vi "Binary Terminal.vi"() -> ()   [LabVIEW 2019]
uses:
  <vilib>/Instr/_visa.llb/VISA Configure Serial Port (Instr).vi
panel:
  in  "Value":dbl=10.0
  in  "CMD":u8(ring) items=["Request Data"=0, "Set Max"=2, "Set Min"=3]
  in  "Send":bool
  out "Chart":dbl(graph)
  out "error out":errorcluster
  in  "stop":bool
  in  "VISA resource name":refnum<visa-resource-name>
  # "To test this code, use a NULL Modem cable and use Binary Instrument.vi to act as the instrument"
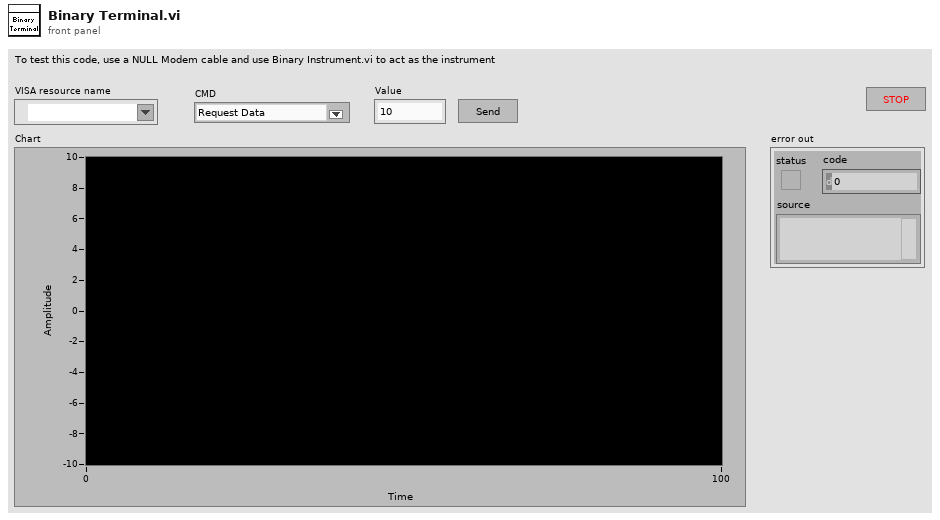
[diagram p1: front panel]
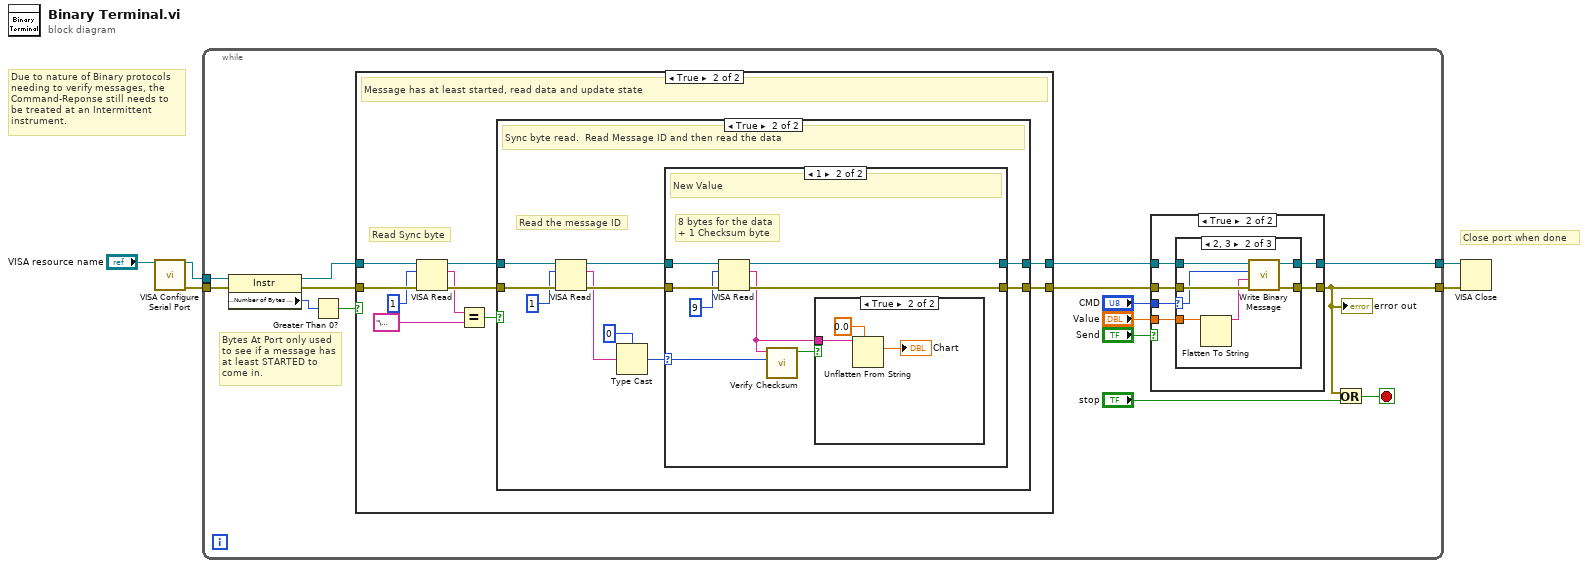
[diagram p0: block diagram]
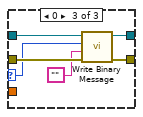
[diagram p4: hidden frame]
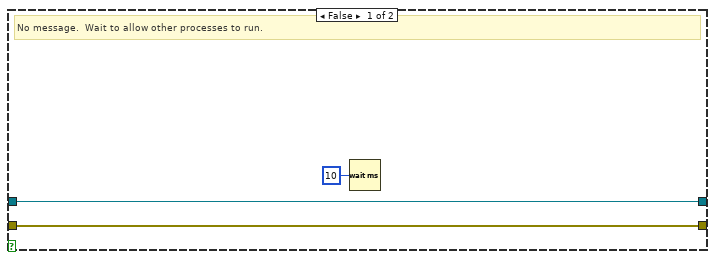
[diagram p5: hidden frame]
diagram:
  # "Due to nature of Binary protocols\nneeding to verify messages, the\nCommand-Reponse still needs to \nbe treated at an Intermittent\ninstrument."
  # "Close port when done"
  n1 = call-poly "VISA Configure Serial Port"("VISA resource name"="VISA resource name") -> ("VISA resource name out"=w1:refnum<visa-resource-name>, "error out"=w4:errorcluster)  [unwired: 13 in]
  n2 = while {
    tunnel: w4 -> [w20]
    tunnel: w1 -> [w16]
    tunnel: [w7] -> w2
    tunnel: [w18] -> w5
    stop <- w12 stop-if-true
    # "Bytes At Port only used\nto see if a message has\nat least STARTED to\ncome in."
    n3 = property class="Instr"(reference=w16, error in=w20) -> (reference out=w13:refnum<visa-resource-name>, error out=w19:errorcluster, "Serial Settings:Number of Bytes at Serial Port"=w15:u32)
    n4 = Greater Than 0?(x=w15) -> (x > 0?=w14:bool)
    n5 = case shown="True" w14 {
      tunnel: w19 -> [w46 w56]
      tunnel: w13 -> [w45 w53]
      tunnel: [w45 w47] -> w6
      tunnel: [w46 w54] -> w17
      frame False {
        # "No message.  Wait to allow other processes to run."
        n6 = Wait (ms)(milliseconds to wait=u32 10) -> ()  [unwired: 1 out]
      }
      frame True {
        # "Read Sync byte"
        # "Message has at least started, read data and update state"
        n7 = VISA Read(VISA resource name=w53, byte count=u32 1, error in (no error)=w56) -> (VISA resource name out=w49:refnum<visa-resource-name>, read buffer=w48:string, error out=w55:errorcluster)  [unwired: 1 out]
        n8 = Equal?(x=w48, y="\u0002") -> (x = y?=w50:bool)
        n9 = case shown="True" w50 {
          tunnel: w49 -> [w57 w64]
          tunnel: w55 -> [w58 w68]
          tunnel: [w57 w59] -> w47
          tunnel: [w58 w66] -> w54
          frame False {
            # "Sync byte was not read.  Ignore the data assuming we are in the middle of a message."
          }
          frame True {
            # "Read the message ID"
            # "Sync byte read.  Read Message ID and then read the data"
            n10 = VISA Read(VISA resource name=w64, byte count=u32 1, error in (no error)=w68) -> (VISA resource name out=w60:refnum<visa-resource-name>, read buffer=w63:string, error out=w67:errorcluster)  [unwired: 1 out]
            n11 = Type Cast(type=u8 0, x=w63) -> (*(type *) &x=w61:u8)
            n12 = case shown="1" w61 {
              selector: w61 -> [_ w72]
              tunnel: w67 -> [w70 w78]
              tunnel: w60 -> [w69 w76]
              tunnel: [w69 w74] -> w59
              tunnel: [w70 w77] -> w66
              frame Default {
                # "Unknown ID.  Ignore the data"
              }
              frame 1 {
                # "8 bytes for the data\n+ 1 Checksum byte"
                # "New Value"
                n13 = VISA Read(VISA resource name=w76, byte count=u32 9, error in (no error)=w78) -> (VISA resource name out=w74:refnum<visa-resource-name>, read buffer=w71:string, error out=w77:errorcluster)  [unwired: 1 out]
                n14 = call "Verify Checksum.vi"("Message ID"=w72, "Data + Checksum"=w71) -> ("Pass"=w73:bool)  [unwired: 9 in]
                n15 = case shown="True" w73 {
                  tunnel: w71 -> [_ w81]
                  frame False {
                  }
                  frame True {
                    n16 = Unflatten From String(type=0.0, binary string=w81) -> (value=→"Chart":dbl)  [unwired: 3 in, 2 out]
                  }
                }
              }
            }
          }
        }
      }
    }
    n17 = case shown="True" "Send" {
      tunnel: w6 -> [w21 w26]
      tunnel: [w21 w25] -> w7
      tunnel: [w22 w28] -> w18
      tunnel: w17 -> [w22 w27]
      tunnel: "Value" -> [_ w23]
      tunnel: "CMD" -> [_ w24]
      frame False {
      }
      frame True {
        n18 = case shown="2, 3" w24 {
          selector: w24 -> [_ w33 w39]
          tunnel: w26 -> [w29 w35 w41]
          tunnel: [w29 w34 w40] -> w25
          tunnel: [w30 w37 w43] -> w28
          tunnel: w27 -> [w30 w36 w42]
          tunnel: w23 -> [_ w32 _]
          frame Default {
          }
          frame 2, 3 {
            n19 = Flatten To String(anything=w32) -> (data string=w31:string)  [unwired: 3 in, 2 out]
            n20 = call "Write Binary Message.vi"("error in"=w36, "Flattened Data"=w31, "Message ID"=w33, "VISA resource in"=w35) -> ("error out"=w37:errorcluster, "VISA resource out"=w34:refnum<visa-resource-name>)  [unwired: 6 in]
          }
          frame 0 {
            n21 = call "Write Binary Message.vi"("error in"=w42, "Flattened Data"="", "Message ID"=w39, "VISA resource in"=w41) -> ("error out"=w43:errorcluster, "VISA resource out"=w40:refnum<visa-resource-name>)  [unwired: 6 in]
          }
        }
      }
    }
    "error out" <- w18
    n22 = Or(x=w18, y="stop") -> (x .or. y?=w12:bool)
  }
  n23 = VISA Close(VISA resource name=w2, error in (no error)=w5) -> ()  [unwired: 1 out]
